vi "OMV_Python.vi"(8 "error in (no error)":errorcluster, 10 "Script":string, 11 "VISA Refnum in":refnum<visa-resource-name>) -> (0 "error out":errorcluster, 3 "VISA Refnum out":refnum<visa-resource-name>)   [LabVIEW 2016]
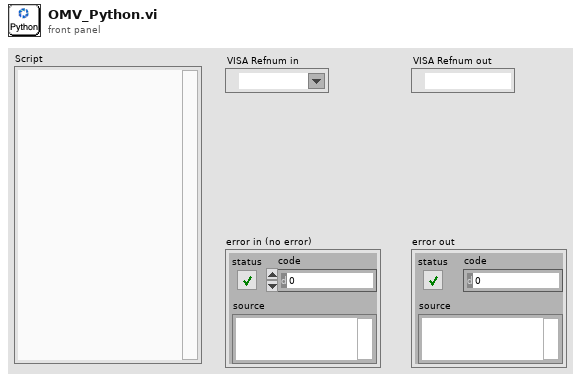
[diagram p1: front panel]
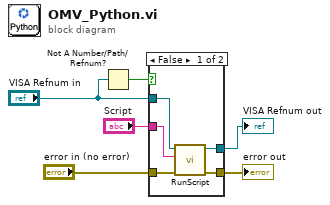
[diagram p0: block diagram]
diagram:
  n1 = Not A Number/Path/Refnum?(number/path/refnum="VISA Refnum in") -> (NaN/Path/Refnum?=w1:bool)
  n2 = case shown="False" w1 {
    tunnel: [w11 w13] -> w6
    tunnel: [w10 w12] -> w5
    tunnel: "Script" -> [w9 _]
    tunnel: "error in (no error)" -> [w8 w12]
    tunnel: "VISA Refnum in" -> [w7 w13]
    frame False {
      n3 = call "RunScript.vi"("error in"=w8, "script"=w9, "VISA Refnum in"=w7) -> ("error out"=w10:errorcluster, "VISA Refnum out"=w11:refnum<visa-resource-name>)  [unwired: 6 in, 1 out]
    }
    frame True {
    }
  }
  "VISA Refnum out" <- w6
  "error out" <- w5
